vi "FGVHysteresisCompensation.vi"(7 "Enum":T2, 8 "error in":errorcluster, 9 "HysteresisSlowIn":T1 {"PolynomCoeff" format="%#.4g"}, 10 "HysteresisFastIn":T1 {"PolynomCoeff" format="%#.4g"}) -> (0 "error out":errorcluster, 1 "HysteresisSlowOut":T1 {"PolynomCoeff" format="%#.4g"}, 2 "HysteresisFastOut":T1 {"PolynomCoeff" format="%#.4g"})   [LabVIEW 2016]
uses:
  controls/Enum.ctl
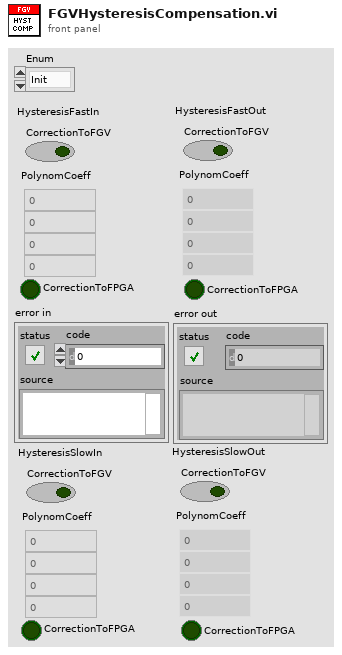
[diagram p1: front panel]
types:
  T1 = cluster{"CorrectionToFGV":bool, "PolynomCoeff":dbl[], "CorrectionToFPGA":bool}
  T2 = typedef "Enum.ctl" = enum16{"Init", "Read", "Write"}
  T3 = cluster{"Correction?":bool, "SlowHS":dbl[], "CorrectionToFPGA":bool}
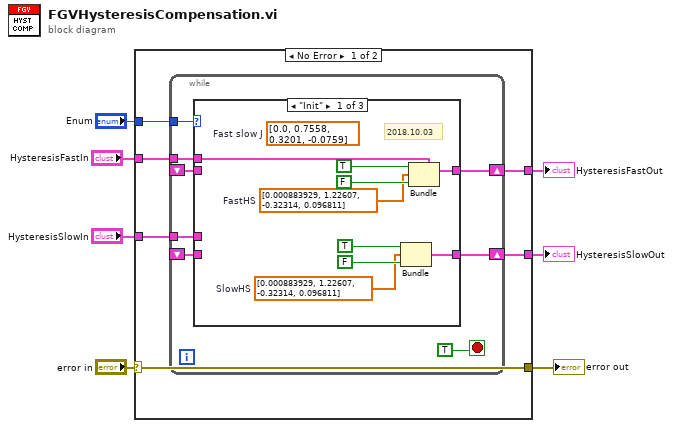
[diagram p0: block diagram]
diagram:
  n1 = case shown="No Error" "error in" {
    selector: "error in" -> [w12 w37]
    tunnel: "Enum" -> [w13 _]
    tunnel: [w12 w37] -> w6
    tunnel: "HysteresisFastIn" -> [w11 w36]
    tunnel: [w10 w36] -> w3
    tunnel: "HysteresisSlowIn" -> [w9 w35]
    tunnel: [w8 w35] -> w1
    frame No Error {
      n2 = while {
        tunnel: w13 -> [w20]
        tunnel: w11 -> [w19]
        shift-right: [w18] -> w10
        shift-left: _ -> [w17]
        tunnel: w9 -> [w16]
        shift-right: [w15] -> w8
        shift-left: _ -> [w14]
        stop <- TRUE stop-if-true
        n3 = case shown="\"Init\"" w20 {
          tunnel: w19 -> [w29 _ w34]
          tunnel: [w30 w32 w34] -> w18
          tunnel: w17 -> [_ w32 _]
          tunnel: w16 -> [_ _ w33]
          tunnel: [w24 w31 w33] -> w15
          tunnel: w14 -> [_ w31 _]
          frame "Init" {
            (unwired) dbl[] [0.0, 0.7558, 0.3201, -0.0759]  # Fast slow J
            w22 = dbl[] [0.000883929, 1.22607, -0.32314, 0.096811]  # SlowHS
            w23 = dbl[] [0.000883929, 1.22607, -0.32314, 0.096811]  # FastHS
            # "2018.10.03"
            n4 = Bundle("Correction?"=TRUE, "SlowHS"=w22, "CorrectionToFPGA"=FALSE) -> (w24:T3)  [unwired: 1 in]
            n5 = Bundle(cluster=w29, "CorrectionToFGV"=TRUE ("Correction?"), "PolynomCoeff"=w23, "CorrectionToFPGA"=FALSE) -> (w30:T1)
          }
          frame "Read", Default {
          }
          frame "Write" {
          }
        }
      }
    }
    frame Error {
    }
  }
  "error out" <- w6
  "HysteresisFastOut" <- w3
  "HysteresisSlowOut" <- w1
